vi "Get Page Properties as Cluster.vi"(8 "error in":errorcluster, 10 "Variant Cluster":variant, 11 "custom device ref in":T1 format="%.0x") -> (0 "error out":errorcluster, 2 "data":variant, 3 "custom device ref out":T1 format="%.0x")   [LabVIEW 2020, in "AIM ARINC 664 Scripting.lvlib"]
uses:
  AIM ARINC 664 Scripting.lvlib
  <vilib>/NI VeriStand/Custom Device API/Custom Device Item Ref.ctl
  <vilib>/NI VeriStand/Custom Device API/Get Item Property (U32).vi
  <vilib>/NI VeriStand/Custom Device API/Get Item Property (I32).vi
  <vilib>/NI VeriStand/Custom Device API/Get Item Property (Boolean).vi
  <vilib>/NI VeriStand/Custom Device API/Get Item Property (String).vi
  <vilib>/NI VeriStand/Custom Device API/Get Item Property (Path).vi
  <vilib>/Utility/Data Type/NI_Data Type.lvlib
  <vilib>/NI VeriStand/Custom Device API/Custom Device API.lvlib
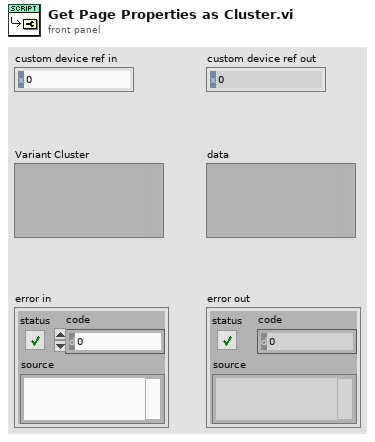
[diagram p1: front panel]
types:
  T1 = typedef "Custom Device API.lvlib/Custom Device Item Ref.ctl" = u64
  T2 = typedef "NI_Data Type.lvlib/Data Type.ctl" = enum8{"Invalid Type", "Void", "I8", "I16", "I32", "I64", "U8", "U16", "U32", "U64", "Single Float", "Double Float", "Extended Float", "Single Complex", "Double Complex", "Extended Complex", "Enum U8", "Enum U16", "Enum U32", "Enum U64", "Single Float With Unit", "Double Float With Unit", "Extended Float With Unit", "Single Complex with Unit", "Double Complex with Unit", "Extended Complex with Unit", "Boolean", "String", "Path", "Picture", "Tag", "Array", "Cluster", "Variant", "LV Variant", "Waveform", "Timestamp", "Digital Waveform", "Digital Data", "ExpressData", "Refnum", "External Data", "VI", "Poly VI", "LabVIEW Class Instance", "Fixed Point", "Set Collection", "Map Collection"}
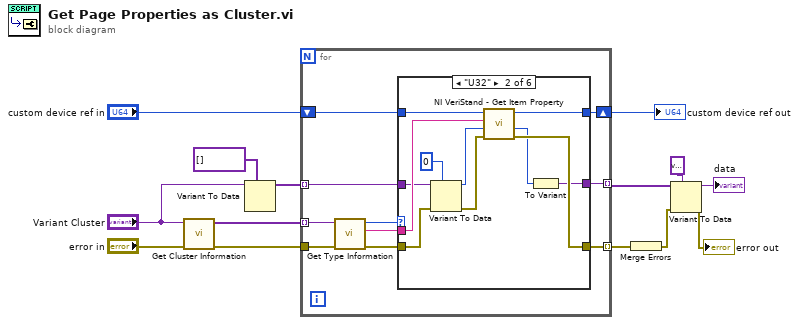
[diagram p0: block diagram]
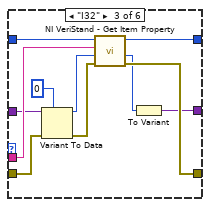
[diagram p3: hidden frame]
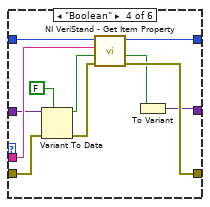
[diagram p4: hidden frame]
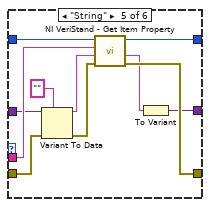
[diagram p5: hidden frame]
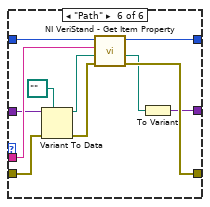
[diagram p6: hidden frame]
diagram:
  n1 = call <vilib>:"Get Cluster Information.vi"("error in (no error)"="error in", "variant"="Variant Cluster") -> ("error out"=w9:errorcluster, "cluster elements"=w10:variant[])  [unwired: 8 in]
  n2 = Variant To Data(type=variant[] [], Variant="Variant Cluster") -> (data=w8:variant[])  [unwired: 1 in, 1 out]
  n3 = for {
    tunnel: w10 -> [w24] mode=indexing
    shift-right: [w20] -> w12
    shift-left: "custom device ref in" -> [w21]
    tunnel: w8 -> [w16] mode=indexing
    tunnel: w9 -> [w23]
    tunnel: [w17] -> w13 mode=indexing
    tunnel: [w15] -> w4 mode=indexing
    n4 = call <vilib>:"Get Type Information.vi"("error in (no error)"=w23, "variant"=w24) -> ("error out"=w18:errorcluster, "name"=w22:string, "type"=w19:T2)  [unwired: 5 in, 2 out]
    n5 = case shown="\"U32\"" w19 {
      tunnel: w22 -> [_ w38 w49 w60 w71 w82]
      tunnel: w21 -> [w27 w37 w48 w59 w70 w81]
      tunnel: [w27 w36 w47 w58 w69 w80] -> w20
      tunnel: w18 -> [w26 w31 w42 w53 w64 w75]
      tunnel: [w26 w35 w46 w57 w68 w79] -> w17
      tunnel: w16 -> [w25 w34 w45 w56 w67 w78]
      tunnel: [w25 w28 w39 w50 w62 w72] -> w15
      frame "Invalid Type", Default {
      }
      frame "U32" {
        n6 = Variant To Data(error in=w31, type=u32 0, Variant=w34) -> (data=w33:u32, error out=w30:errorcluster)
        n7 = call-poly <vilib>:"NI VeriStand - Get Item Property.vi"("error in (no error)"=w30, "Default Value"=w33, "Property Name"=w38, "Item Ref in"=w37) -> ("error out"=w35:errorcluster, "Value"=w29:u32, "Item Ref out"=w36:T1)  [unwired: 4 in, 1 out]
        n8 = To Variant(anything=w29) -> (Variant=w28:variant)
      }
      frame "I32" {
        n9 = Variant To Data(error in=w42, type=0, Variant=w45) -> (data=w44:i32, error out=w41:errorcluster)
        n10 = call-poly <vilib>:"NI VeriStand - Get Item Property.vi"("error in (no error)"=w41, "Default Value"=w44, "Property Name"=w49, "Item Ref in"=w48) -> ("error out"=w46:errorcluster, "Value"=w40:i32, "Item Ref out"=w47:T1)  [unwired: 4 in, 1 out]
        n11 = To Variant(anything=w40) -> (Variant=w39:variant)
      }
      frame "Boolean" {
        n12 = Variant To Data(error in=w53, type=FALSE, Variant=w56) -> (data=w55:bool, error out=w52:errorcluster)
        n13 = call-poly <vilib>:"NI VeriStand - Get Item Property.vi"("error in (no error)"=w52, "Default Value"=w55, "Property Name"=w60, "Item Ref in"=w59) -> ("error out"=w57:errorcluster, "Value"=w51:bool, "Item Ref out"=w58:T1)  [unwired: 4 in, 1 out]
        n14 = To Variant(anything=w51) -> (Variant=w50:variant)
      }
      frame "String" {
        n15 = Variant To Data(error in=w64, type="", Variant=w67) -> (data=w66:string, error out=w63:errorcluster)
        n16 = call-poly <vilib>:"NI VeriStand - Get Item Property.vi"("error in (no error)"=w63, "Default Value"=w66, "Property Name"=w71, "Item Ref in"=w70) -> ("error out"=w68:errorcluster, "Value"=w61:string, "Item Ref out"=w69:T1)  [unwired: 4 in, 1 out]
        n17 = To Variant(anything=w61) -> (Variant=w62:variant)
      }
      frame "Path" {
        n18 = Variant To Data(error in=w75, type=path "", Variant=w78) -> (data=w77:path, error out=w74:errorcluster)
        n19 = call-poly <vilib>:"NI VeriStand - Get Item Property.vi"("error in (no error)"=w74, "Default Value"=w77, "Property Name"=w82, "Item Ref in"=w81) -> ("error out"=w79:errorcluster, "Value"=w73:path, "Item Ref out"=w80:T1)  [unwired: 4 in, 1 out]
        n20 = To Variant(anything=w73) -> (Variant=w72:variant)
      }
    }
  }
  "custom device ref out" <- w12
  n21 = Merge Errors(w13) -> (w3:errorcluster)
  n22 = Variant To Data(error in=w3, type=variant, Variant=w4) -> (data=→"data":variant, error out=→"error out":errorcluster)
